vi "Sub_Read_Fixed_Header.vi"(8 "error in (no error)":errorcluster, 11 "connection ID":refnum<k5>) -> (0 "error out":errorcluster, 1 "MessageType":T1, 2 "Remaining Length":u32, 3 "connection ID out":refnum<k5>, 5 "QoS Level":T2, 6 "DUP Flag":bool, 7 "RETAIN":bool)   [LabVIEW 2019, in "MQTT_Functions.lvlib"]
uses:
  MQTT_Functions.lvlib
  Controls/QoS.ctl
  Controls/MessageType.ctl
panel:
  # "fixed header"
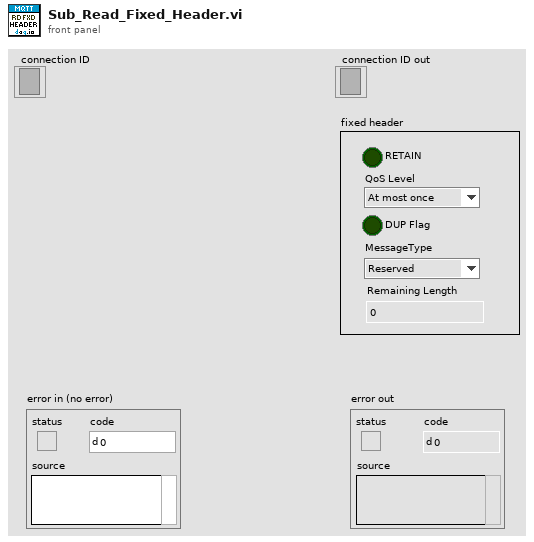
[diagram p1: front panel]
types:
  T1 = typedef "MQTT_Functions.lvlib/MessageType.ctl" = enum32{"Reserved", "CONNECT", "CONNACK", "PUBLISH", "PUBACK", "PUBREC", "PUBREL", "PUBCOMP", "SUBSCRIBE", "SUBACK", "UNSUBSCRIBE", "UNSUBACK", "PINGREQ", "PINGRESP", "DISCONNECT", "Reserved2"}
  T2 = typedef "MQTT_Functions.lvlib/QoS.ctl" = enum8{"At most once", "At least once", "Exactly once", "Reserved"}
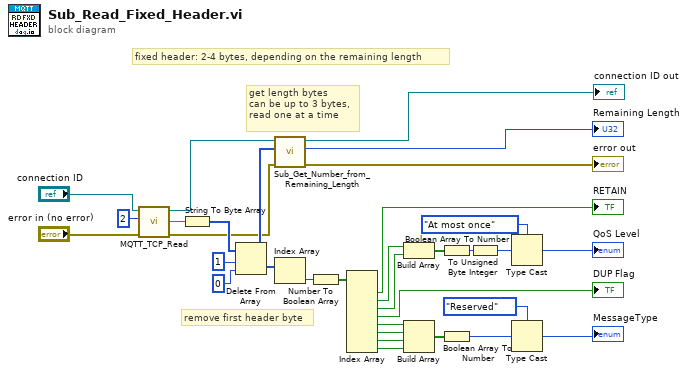
[diagram p0: block diagram]
diagram:
  # "fixed header: 2-4 bytes, depending on the remaining length"
  # "get length bytes\ncan be up to 3 bytes,\nread one at a time"
  # "remove first header byte"
  n1 = call "MQTT_TCP_Read.vi"("error in (no error)"="error in (no error)", "bytes to read"=2, "connection ID"="connection ID") -> ("error out"=w3:errorcluster, "data out"=w5:string, "connection ID out"=w7:refnum<k5>)  [unwired: 6 in]
  n2 = String To Byte Array(string=w5) -> (unsigned byte array=w4:u8[])
  n3 = Delete From Array(array=w4, length=1, index=0) -> (deleted portion=w29:u8[], array with subset deleted=w11:u8[])
  n4 = call "Sub_Get_Number_from_Remaining_Length.vi"("error in (no error)"=w3, "Remaining Length"=w11, "connection ID"=w7) -> ("error out"=→"error out":errorcluster, "X"=→"Remaining Length":u32, "connection ID out"=→"connection ID out":refnum<k5>)  [unwired: 6 in]
  n5 = Index Array(array=w29) -> (element=w28:u8)  [unwired: 1 in]
  n6 = Number To Boolean Array(number=w28) -> (Boolean array=w27:bool[])
  n7 = Index Array(array=w27) -> (element #1=→"RETAIN":bool, element #2=w25:bool, element #3=w24:bool, element #4=→"DUP Flag":bool, element #5=w20:bool, element #6=w19:bool, element #7=w18:bool, element #8=w17:bool)  [unwired: 8 in]
  n8 = Build Array(w25, w24) -> (w23:bool[])
  n9 = Build Array(w20, w19, w18, w17) -> (w16:bool[])
  n10 = Boolean Array To Number(Boolean array=w23) -> (number=w13:u32)
  n11 = Boolean Array To Number(Boolean array=w16) -> (number=w14:u32)
  n12 = To Unsigned Byte Integer(number=w13) -> (unsigned 8bit integer=w1:u8)
  n13 = Type Cast(type=QoS."At most once" ("QoS 2"), x=w1) -> (*(type *) &x=→"QoS Level":T2)
  n14 = Type Cast(type=MessageType."Reserved" ("MessageType"), x=w14) -> (*(type *) &x=→"MessageType":T1)
